vi "Right Side AutoCorrelation.vi"(0 "Normalized Signal Waveform In":waveform(dbl), 2 "Error In":errorcluster, 3 "Autocorrelation Peak Width":dbl, 4 "Autocorrelation Peak Threshold":dbl, 5 "AutoCorrelation Min Lag":dbl, 7 "AutoCorrelation Max Lag":dbl, 9 "AutoCorrelation Peak Ratio Threshold":dbl) -> (12 "Best Lag":dbl, 13 "Autocorrelation - Right Side":dbl[](array[numeric]), 14 "First Strong Peak Found?":bool, 15 "Max Valid Peak Amplitude":dbl, 16 "Zero Lag Amplitude":dbl, 17 "# Valid Peaks":i32, 18 "First Strong Peak Amplitude":dbl, 19 "Full Autocorrelation Waveform Graph":dbl[](graph), 20 "Valid Peaks Found from AutoCorr?":bool, 21 "Valid Peak Mask?":bool[](array[boolean]), 22 "First Strong Peak Lag":dbl, 23 "Valid AutoCorr Peak Locations":dbl[](array[numeric]), 24 "Periodic Signal?":bool, 25 "Valid AutoCorr Peak Amplitudes":dbl[](array[numeric]), 26 "Error Out":errorcluster, 27 "Right Side AutoCorrelation Waveform Graph":dbl[](graph))   [LabVIEW 2025]
uses:
  <vilib>/Analysis/2dsp.llb/1D Auto Correlation (DBL).vi
  <vilib>/Analysis/NI_AALPro.lvlib
  <vilib>/Analysis/NI_AAL_SigProc.lvlib
panel:
  out "Lag of Max Valid Peak":dbl
  out "Autocorrelation-Full":dbl[](array[numeric])
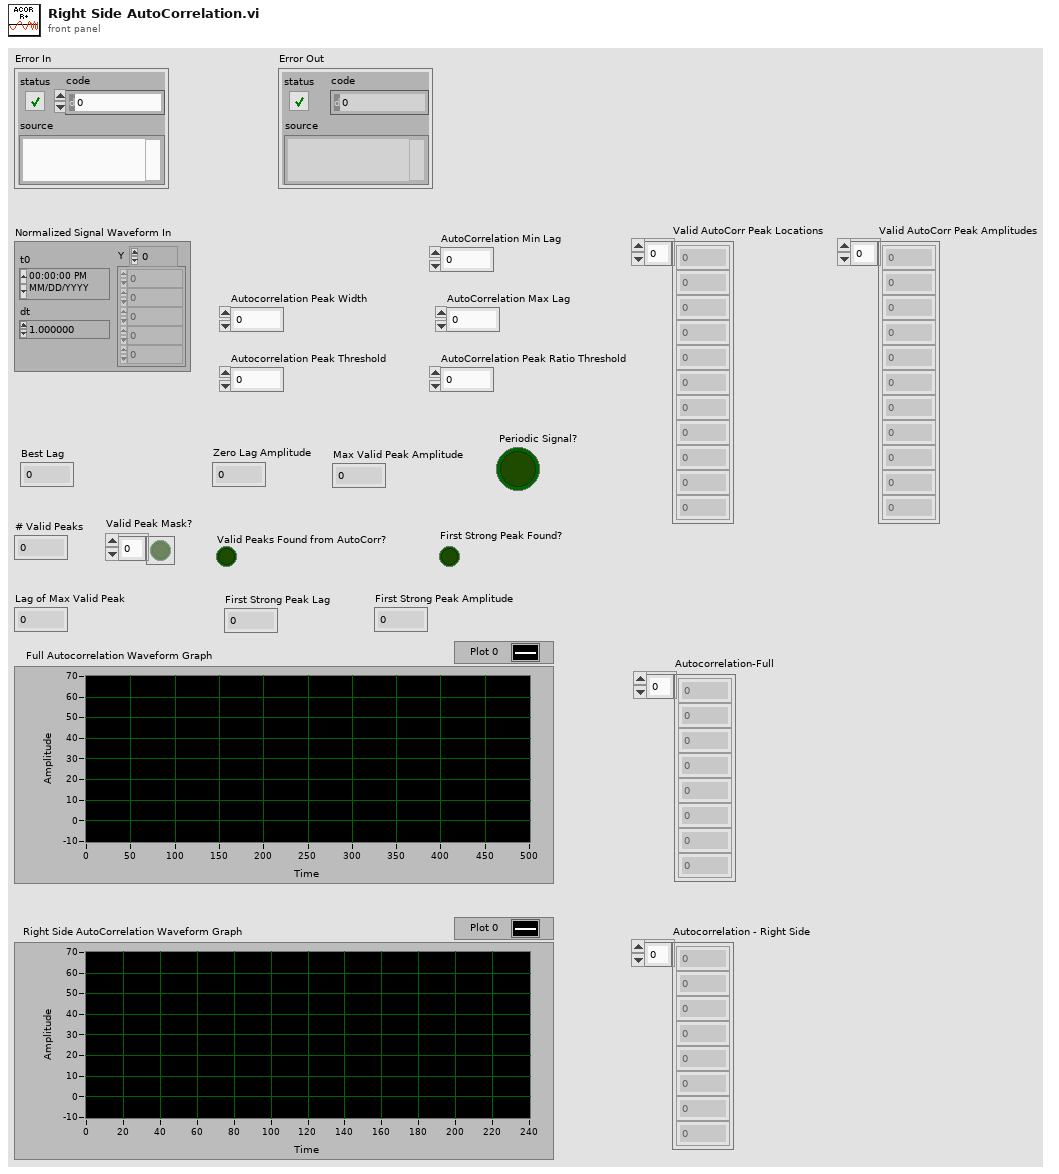
[diagram p1: front panel]
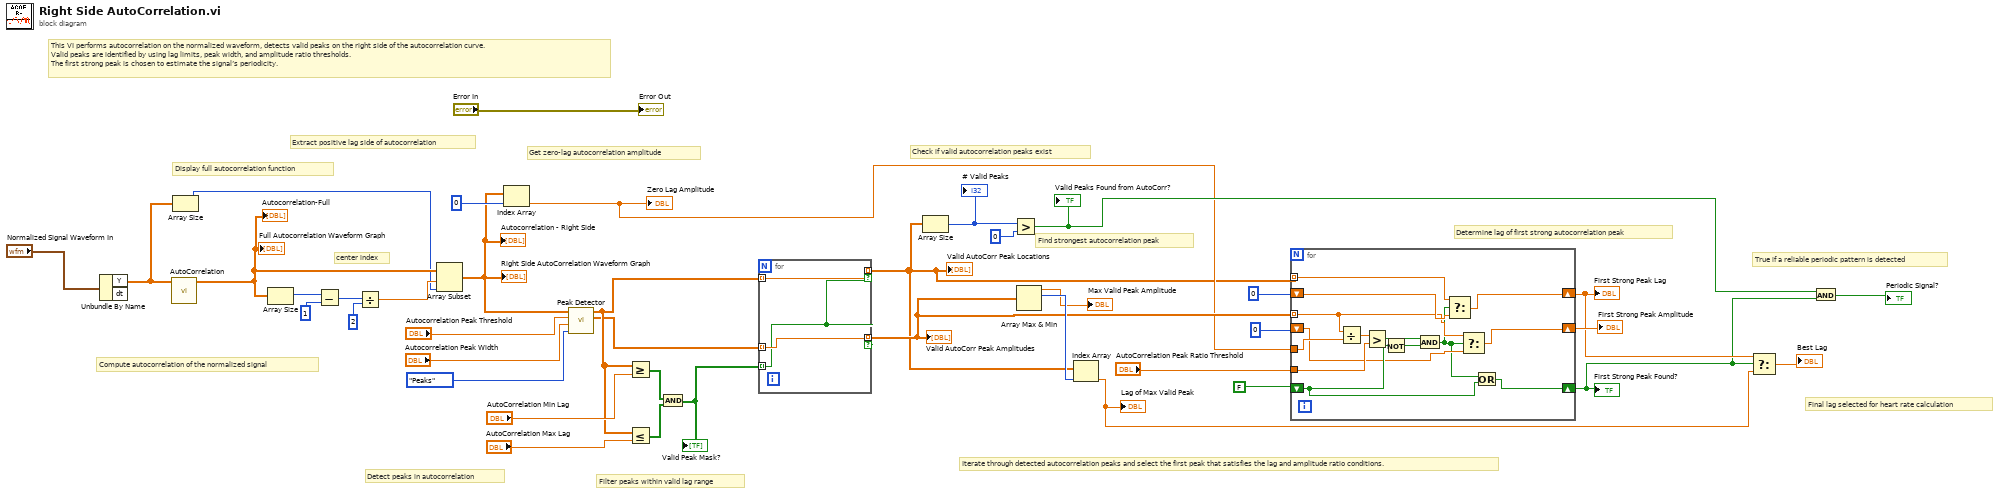
[diagram p0: block diagram]
diagram:
  # "True if a reliable periodic pattern is detected"
  # "Final lag selected for heart rate calculation"
  # "Iterate through detected autocorrelation peaks and select the first peak that satisfies the lag and amplitude ratio conditions."
  # "Determine lag of first strong autocorrelation peak"
  # "Find strongest autocorrelation peak"
  # "Check if valid autocorrelation peaks exist"
  # "Extract positive lag side of autocorrelation"
  # "Filter peaks within valid lag range"
  # "Detect peaks in autocorrelation"
  # "Get zero-lag autocorrelation amplitude"
  # "Display full autocorrelation function"
  # "Compute autocorrelation of the normalized signal"
  # "This VI performs autocorrelation on the normalized waveform, detects valid peaks on the right side of the autocorrelation curve. \nValid peaks are identified by using lag limits, peak width, and amplitude ratio thresholds. \nThe first strong peak is chosen to estimate the signal’s periodicity."
  # "center index"
  n1 = Unbundle By Name("Normalized Signal Waveform In") -> ("Y"=w32:dbl[])  [unwired: 1 out]
  n2 = call-poly <vilib>:"AutoCorrelation.vi"("X"=w32) -> ("Rxx"=w34:dbl[])  [unwired: 9 in, 1 out]
  "Full Autocorrelation Waveform Graph" <- w34
  "Autocorrelation-Full" <- w34
  n3 = Array Size(array=w32) -> (size(s)=w31:i32)
  n4 = Array Size(array=w34) -> (size(s)=w39:i32)
  n5 = Subtract(x=w39, y=1) -> (x-y=w37:i32)
  n6 = Divide(x=w37, y=2) -> (x/y=w35:dbl)
  n7 = Array Subset(array=w34, index=w35, length=w31) -> (w30:dbl[])
  "Right Side AutoCorrelation Waveform Graph" <- w30
  "Autocorrelation - Right Side" <- w30
  n8 = Index Array(array=w30, index=0) -> (element=w11:dbl)
  "Zero Lag Amplitude" <- w11
  n9 = call <vilib>:"Peak Detector.vi"("peaks/valleys"=enum32{"Peaks", "Valleys"}."Peaks", "width"="Autocorrelation Peak Width", "threshold"="Autocorrelation Peak Threshold", "X"=w30) -> ("Amplitudes"=w21:dbl[], "Locations"=w22:dbl[])  [unwired: 3 in, 3 out]
  n10 = Greater Or Equal?(x=w22, y="AutoCorrelation Min Lag") -> (x >= y?=w24:bool[])
  n11 = Less Or Equal?(x=w22, y="AutoCorrelation Max Lag") -> (x <= y?=w23:bool[])
  n12 = And(x=w24, y=w23) -> (x .and. y?=w20:bool[])
  "Valid Peak Mask?" <- w20
  n13 = for {
    tunnel: w22 -> [w43] mode=indexing
    tunnel: w21 -> [w42] mode=indexing
    tunnel: w20 -> [w41] mode=indexing
    tunnel: [w43] -> w9 mode=indexing if=w41
    tunnel: [w42] -> w12 mode=indexing if=w41
  }
  "Valid AutoCorr Peak Locations" <- w9
  "Valid AutoCorr Peak Amplitudes" <- w12
  n14 = Array Size(array=w9) -> (size(s)=w19:i32)
  "# Valid Peaks" <- w19
  n15 = Greater?(x=w19, y=0) -> (0:w15:bool)
  "Valid Peaks Found from AutoCorr?" <- w15
  n16 = Array Max & Min(array=w12) -> (max value=→"Max Valid Peak Amplitude":dbl, max index (indices)=w17:i32)  [unwired: 2 out]
  n17 = Index Array(array=w9, index=w17) -> (element=w3:dbl)
  "Lag of Max Valid Peak" <- w3
  n18 = for {
    tunnel: w12 -> [w48] mode=indexing
    tunnel: w9 -> [w51] mode=indexing
    tunnel: w11 -> [w57]
    tunnel: "AutoCorrelation Peak Ratio Threshold" -> [w56]
    shift-right: [w49] -> w4
    shift-left: 0 -> [w50]
    shift-right: [w46] -> w5
    shift-left: 0 -> [w47]
    shift-right: [w52] -> w1
    shift-left: FALSE -> [w53]
    n19 = Divide(x=w48, y=w57) -> (x/y=w45:dbl)
    n20 = Greater?(x=w45, y=w56) -> (0:w54:bool)
    n21 = Not(x=w53) -> (.not. x?=w55:bool)
    n22 = And(x=w54, y=w55) -> (x .and. y?=w44:bool)
    n23 = Select(t=w51, s=w44, f=w50) -> (s? t:f=w49:dbl)
    n24 = Select(t=w48, s=w44, f=w47) -> (s? t:f=w46:dbl)
    n25 = Or(x=w44, y=w53) -> (x .or. y?=w52:bool)
  }
  "First Strong Peak Lag" <- w4
  "First Strong Peak Amplitude" <- w5
  "First Strong Peak Found?" <- w1
  n26 = Select(t=w4, s=w1, f=w3) -> (s? t:f=→"Best Lag":dbl)
  n27 = And(x=w15, y=w1) -> (x .and. y?=→"Periodic Signal?":bool)
  "Error Out" <- "Error In"
